vi "CSV Read.vi"() -> ()   [LabVIEW 2016]
panel:
  out "Diluent MF":string
  out "Fuel Used":dbl[unit] format="%_6g"
  out "Oxidizer Used":dbl[unit] format="%_6g"
  out "Diluent Used":dbl[unit] format="%_6g"
  out "Predicted CJ Speed":dbl[unit]
  out "Equivalence Ratio":string
  out "Test Number":string
  out "Diluent Cutoff":dbl[unit]
  out "Oxidizer Cutoff":dbl[unit]
  out "Fuel Cutoff":dbl[unit]
  in  "CSV In":string[][](array[string])
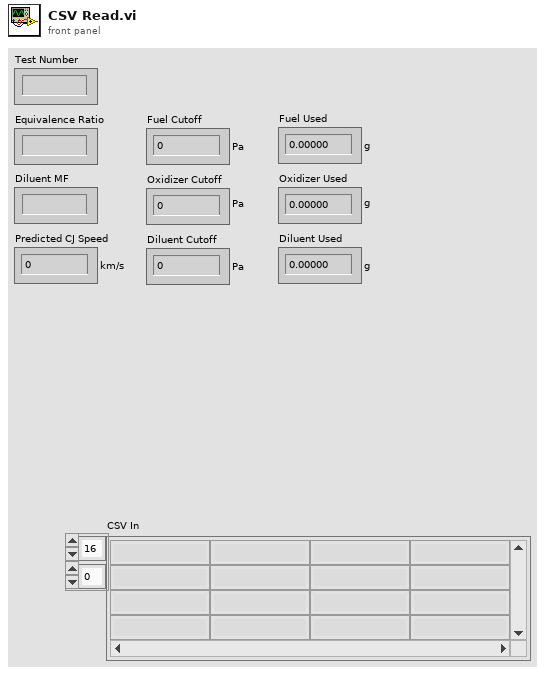
[diagram p1: front panel]
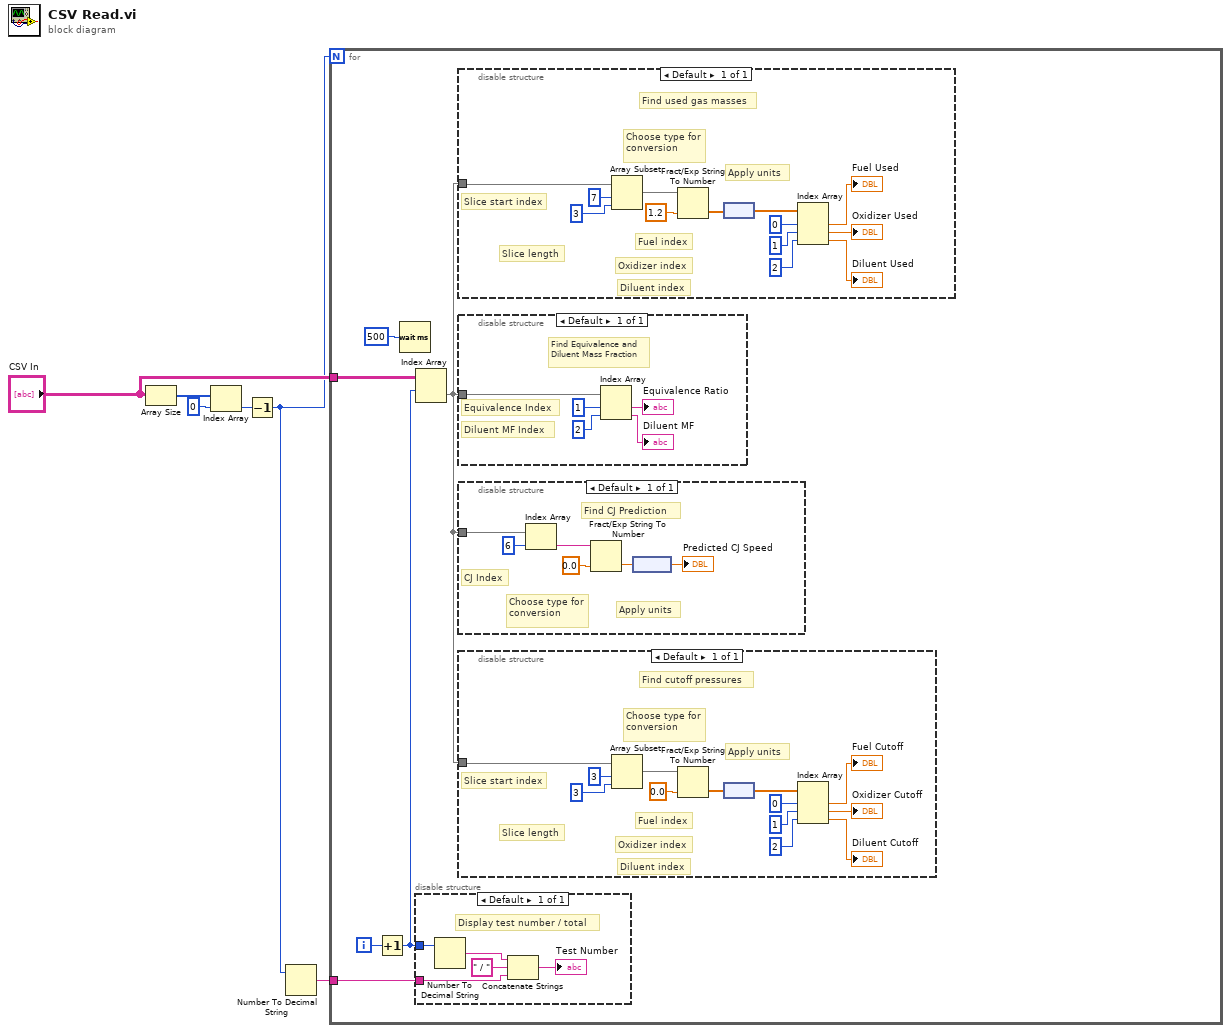
[diagram p0: block diagram]
diagram:
  n1 = Array Size(array="CSV In") -> (size(s)=w6:i32[])
  n2 = Index Array(array=w6, index=0) -> (element=w4:i32)
  n3 = Decrement(x=w4) -> (x-1=w2:i32)
  n4 = Number To Decimal String(number=w2) -> (decimal integer string=w1:string)  [unwired: 1 in]
  n5 = for {
    N: w2 -> [_]
    tunnel: "CSV In" -> [w10]
    tunnel: w1 -> [w9]
    i -> [w12]
    n6 = Increment(x=w12) -> (x+1=w8:i32)
    n7 = Wait (ms)(milliseconds to wait=u32 500) -> ()  [unwired: 1 out]
    n8 = Index Array(array=w10, index (row)=w8) -> (element=w7:string[])  [unwired: 1 in]
    n9 = disable-structure shown="Default" {
      disable-tunnel: w9 -> [w52]
      disable-tunnel: w8 -> [w50]
      frame Enabled {
        # "Display test number / total"
        n10 = Number To Decimal String(number=w50) -> (decimal integer string=w51:string)  [unwired: 1 in]
        n11 = Concatenate Strings(w51, " / " ("string"), w52) -> (→"Test Number":string)
      }
    }
    n12 = disable-structure shown="Default" {
      disable-tunnel: w7 -> [w18]
      frame Enabled {
        # "Find used gas masses"
        # "Slice start index"
        # "Slice length"
        # "Choose type for conversion"
        # "Apply units"
        # "Diluent index"
        # "Oxidizer index"
        # "Fuel index"
        n13 = Array Subset(array=w18, index=7, length=3) -> (w16:string[])
        n14 = Fract/Exp String To Number(string=w16, default (0 dbl)=1.2 ("default (0 I32)")) -> (number=w14:dbl[])  [unwired: 2 in, 1 out]
        n15 = node(w14) -> (w13:dbl[unit][])
        n16 = Index Array(array=w13, index #1=0 ("index"), index #2=1 ("index"), index #3=2 ("index")) -> (element #1=→"Fuel Used":dbl[unit], element #2=→"Oxidizer Used":dbl[unit], element #3=→"Diluent Used":dbl[unit])
      }
    }
    n17 = disable-structure shown="Default" {
      disable-tunnel: w7 -> [w28]
      frame Enabled {
        # "Diluent MF Index"
        # "Find Equivalence and Diluent Mass Fraction"
        # "Equivalence Index"
        n18 = Index Array(array=w28, index #1=1 ("index"), index #2=2 ("index")) -> (element #1=→"Equivalence Ratio":string, element #2=→"Diluent MF":string)
      }
    }
    n19 = disable-structure shown="Default" {
      disable-tunnel: w7 -> [w35]
      frame Enabled {
        # "Apply units"
        # "Choose type for conversion"
        # "CJ Index"
        # "Find CJ Prediction"
        n20 = Index Array(array=w35, index=6) -> (element=w34:string)
        n21 = Fract/Exp String To Number(string=w34, default (0 dbl)=0.0 ("default (0 I32)")) -> (number=w33:dbl)  [unwired: 2 in, 1 out]
        n22 = node(w33) -> (→"Predicted CJ Speed":dbl[unit])
      }
    }
    n23 = disable-structure shown="Default" {
      disable-tunnel: w7 -> [w39]
      frame Enabled {
        # "Find cutoff pressures"
        # "Slice start index"
        # "Slice length"
        # "Choose type for conversion"
        # "Apply units"
        # "Diluent index"
        # "Oxidizer index"
        # "Fuel index"
        n24 = Array Subset(array=w39, index=3, length=3) -> (w49:string[])
        n25 = Fract/Exp String To Number(string=w49, default (0 dbl)=0.0 ("default (0 I32)")) -> (number=w47:dbl[])  [unwired: 2 in, 1 out]
        n26 = node(w47) -> (w43:dbl[unit][])
        n27 = Index Array(array=w43, index #1=0 ("index"), index #2=1 ("index"), index #3=2 ("index")) -> (element #1=→"Fuel Cutoff":dbl[unit], element #2=→"Oxidizer Cutoff":dbl[unit], element #3=→"Diluent Cutoff":dbl[unit])
      }
    }
  }
